vi "Send VISA Query.vi"(8 "error in (no error)":errorcluster, 10 "Command":string, 11 "336XX in":refnum<class "336XX.lvclass">) -> (0 "error out":errorcluster, 2 "Response":string, 3 "336XX out":refnum<class "336XX.lvclass">)   [LabVIEW 2019, in "336XX.lvlib" / "336XX.lvclass"]
uses:
  Library/336XX.lvclass
  Library/336XX.lvclass/336XX.ctl
  <instrlib>/Agilent 3352X Series/Agilent 3352X Series.lvlib
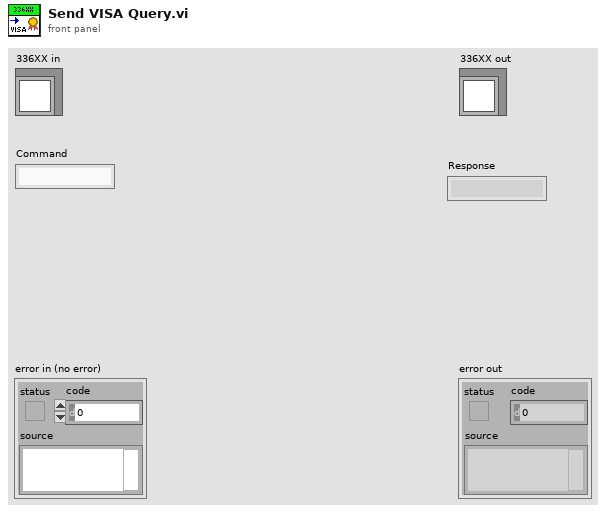
[diagram p1: front panel]
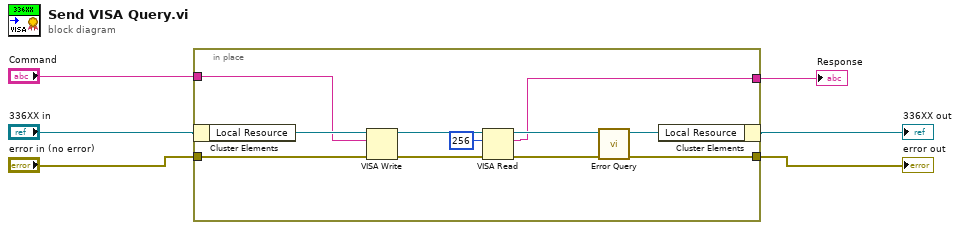
[diagram p0: block diagram]
diagram:
  n1 = in-place {
    in-place-border: "error in (no error)" -> [w14]
    in-place-border: [w13] -> w3
    in-place-border: "Command" -> [w12]
    in-place-border: [w8] -> w1
    n2 = in-place-cluster #1("336XX in") -> ("Local Resource"=w16:refnum<visa-resource-name>)
    n3 = VISA Write(VISA resource name=w16, write buffer=w12, error in (no error)=w14) -> (VISA resource name out=w10:refnum<visa-resource-name>, error out=w15:errorcluster)  [unwired: 1 out]
    n4 = VISA Read(VISA resource name=w10, byte count=u32 256, error in (no error)=w15) -> (VISA resource name out=w9:refnum<visa-resource-name>, read buffer=w8:string, error out=w11:errorcluster)  [unwired: 1 out]
    n5 = call <instrlib>:"Error Query.vi"("error in (no error)"=w11, "VISA resource name"=w9) -> ("error out"=w13:errorcluster, "VISA resource name out"=w17:refnum<visa-resource-name>)  [unwired: 8 out]
    n6 = in-place-cluster #1("Local Resource"=w17) -> (→"336XX out":refnum<class "336XX.lvclass">)
  }
  "error out" <- w3
  "Response" <- w1
